vi "Set All Attributes.vi"(8 "error in":errorcluster, 10 "Section Node":refnum<k20>, 11 "Section Ref in":refnum<data-value>) -> (0 "error out":errorcluster, 3 "Section Ref out":refnum<data-value>)   [LabVIEW 2024, in "Config File Parser.lvlib" / "Section.lvclass"]
uses:
  Section.lvclass
  Section.lvclass/Section.ctl
  <vilib>/xml/Close Reference(Node).vi
  <resource>/objmgr/DOMUserDefRef.rc
  <vilib>/xml/NI_XML.lvlib
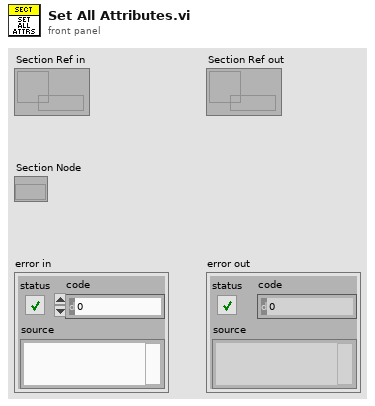
[diagram p1: front panel]
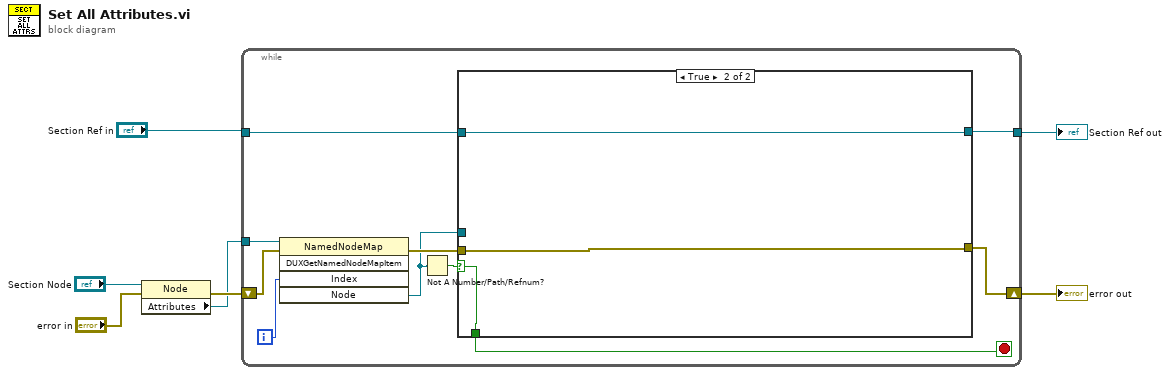
[diagram p0: block diagram]
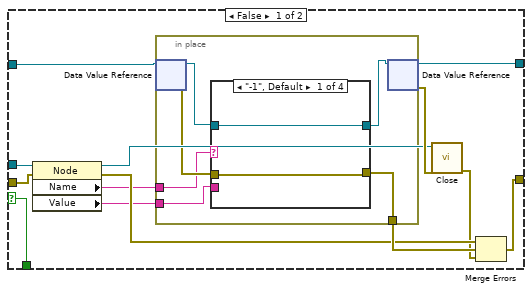
[diagram p2: hidden frame]
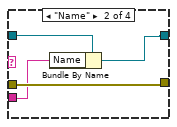
[diagram p3: hidden frame]
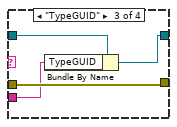
[diagram p4: hidden frame]
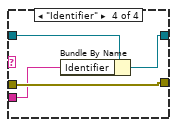
[diagram p5: hidden frame]
diagram:
  n1 = property on="Property Node" class="Node"(reference="Section Node", error in="error in") -> (error out=w6:errorcluster, "Attributes"=w3:refnum<k20>)  [unwired: 1 out]
  n2 = while {
    tunnel: w3 -> [w14]
    shift-right: [w15] -> w5
    shift-left: w6 -> [w17]
    tunnel: "Section Ref in" -> [w10]
    tunnel: [w11] -> w1
    i -> [w9]
    stop <- w8 stop-if-true
    n3 = invoke on="Invoke Node" class="NamedNodeMap" method="DUXGetNamedNodeMapItem"(reference=w14, error in=w17, "Index"=w9) -> (error out=w16:errorcluster, "Node"=w12:refnum<k20>)  [unwired: 2 in, 3 out]
    n4 = Not A Number/Path/Refnum?(number/path/refnum=w12) -> (NaN/Path/Refnum?=w13:bool)
    n5 = case shown="True" w13 {
      selector: w13 -> [w19 w51]
      tunnel: w12 -> [w24 _]
      tunnel: w16 -> [w30 w53]
      tunnel: [w28 w53] -> w15
      tunnel: [w21 w52] -> w11
      tunnel: w10 -> [w20 w52]
      tunnel: [w19 w51] -> w8
      frame False {
        n6 = property on="Property Node" class="Node"(reference=w24, error in=w30) -> (reference out=w22:refnum<k20>, error out=w27:errorcluster, "Name"=w23:string, "Value"=w18:string)
        n7 = in-place "In Place Element Structure" {
          in-place-border: w23 -> [w32]
          in-place-border: [w35] -> w29
          in-place-border: w18 -> [w31]
          n8 = in-place-dvr #1(w20) -> (w34:refnum<class "Section.lvclass">, w36:errorcluster)
          n9 = case shown="\"-1\", Default" w32 {
            tunnel: w34 -> [w37 w40 w44 w48]
            tunnel: [w37 w39 w43 w47] -> w33
            tunnel: w31 -> [_ w41 w45 w49]
            tunnel: w36 -> [w38 w42 w46 w50]
            tunnel: [w38 w42 w46 w50] -> w35
            frame "-1", Default {
            }
            frame "Name" {
              n10 = Bundle By Name(cluster=w40, "Name"=w41) -> (w39:refnum<class "Section.lvclass">)
            }
            frame "TypeGUID" {
              n11 = Bundle By Name(cluster=w44, "TypeGUID"=w45) -> (w43:refnum<class "Section.lvclass">)
            }
            frame "Identifier" {
              n12 = Bundle By Name(cluster=w48, "Identifier"=w49) -> (w47:refnum<class "Section.lvclass">)
            }
          }
          n13 = in-place-dvr #1(w33) -> (w21:refnum<data-value>, w26:errorcluster)
        }
        n14 = call-poly <vilib>:"Close.vi"("error in (no error)"=w26, "node"=w22) -> ("error out"=w25:errorcluster)  [unwired: 7 in]
        n15 = Merge Errors(w27, w29, w25) -> (w28:errorcluster)
      }
      frame True {
      }
    }
  }
  "error out" <- w5
  "Section Ref out" <- w1
